vi "Perform Action.vi"(8 "error in (no error)":errorcluster, 10 "Input":variant, 11 "Sample PI Control in":refnum<class "Sample PI Control.lvclass">) -> (0 "error out":errorcluster, 2 "Output":variant, 3 "Sample PI Control out":refnum<class "Sample PI Control.lvclass">)   [LabVIEW 2023, in "Sample PI Control.lvclass"]
uses:
  Sample PI Control.lvclass
  D:/git/HAL/HAL GOOP4/Task/Task Base/Task Base.lvclass
  Task/Task Base/Task Base.lvclass/Task Base.ctl
  <vilib>/Utility/error.llb/Error Cluster From Error Code.vi
  <vilib>/addons/control/pid/pid.llb/PID (DBL).vi
  Sample PI Control.lvclass/Sample PI Control.ctl
  Measure and Stimulus Subsystems/Measure and Stimulus Subsystems.lvclass
  Task/Task Base/Task Base.lvclass
  <vilib>/addons/control/pid/NI_PID_pid.lvlib
panel:
  out "Powersensor Scalar":dbl
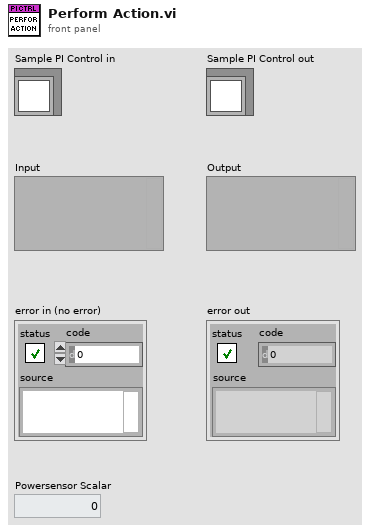
[diagram p1: front panel]
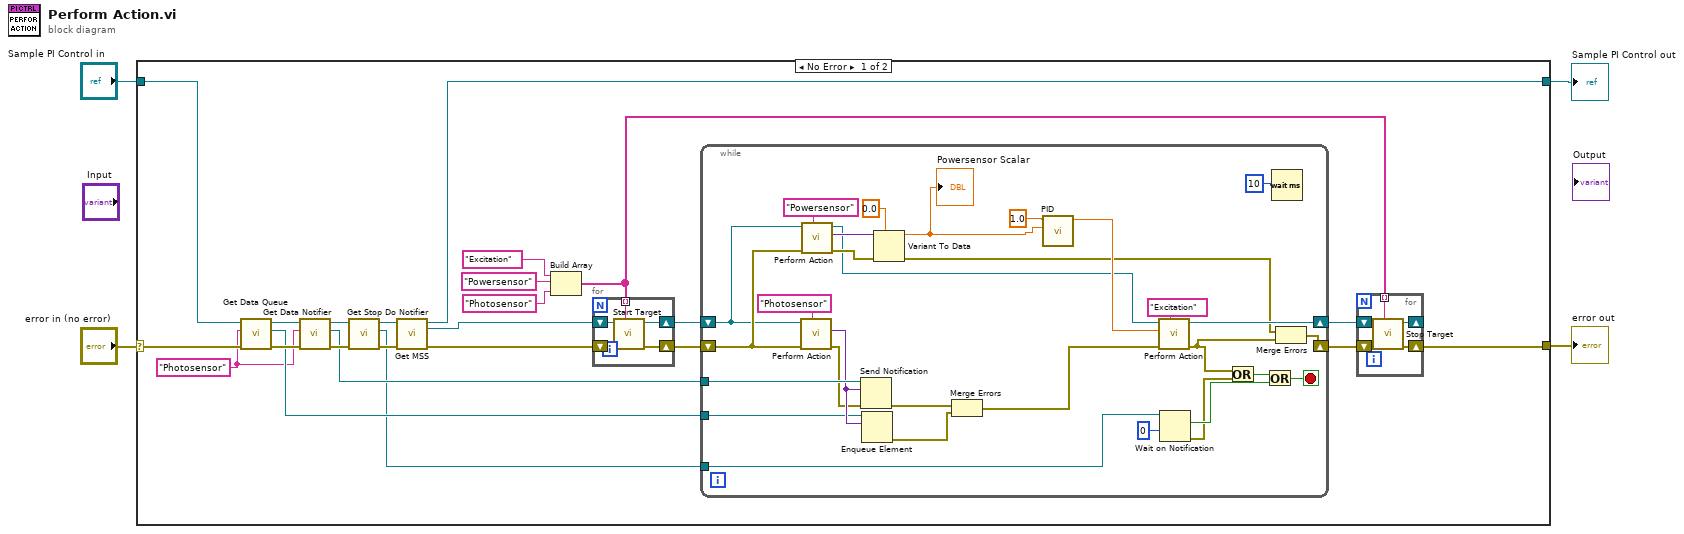
[diagram p0: block diagram]
diagram:
  n1 = case shown="No Error" "error in (no error)" {
    selector: "error in (no error)" -> [w25 w70]
    tunnel: [w21 w70] -> w3
    tunnel: [w11 w69] -> w1
    tunnel: "Sample PI Control in" -> [w13 w69]
    frame No Error {
      w7 = "Photosensor" ("Target Identifier")
      n2 = call "Get Data Queue.vi"("error in (no error)"=w25, "Target Name"=w7, "Task Base in"=w13) -> ("error out"=w14:errorcluster, "Data Queue"=w12:refnum<queue>, "Task Base out"=w9:refnum<class "Sample PI Control.lvclass">)  [unwired: 6 in]
      n3 = call "Get Data Notifier.vi"("error in (no error)"=w14, "Target Name"=w7, "Task Base in"=w9) -> ("error out"=w10:errorcluster, "Data Notifier"=w6:refnum<notifier>, "Task Base out"=w8:refnum<class "Sample PI Control.lvclass">)  [unwired: 6 in]
      n4 = call "Get Stop Do Notifier.vi"("error in (no error)"=w10, "Task Base in"=w8) -> ("error out"=w20:errorcluster, "Stop Do"=w5:refnum<notifier>, "Task Base out"=w19:refnum<class "Sample PI Control.lvclass">)  [unwired: 7 in]
      n5 = call "Get MSS.vi"("error in (no error)"=w20, "Task Base in"=w19) -> ("error out"=w24:errorcluster, "MSS"=w23:refnum<class "Measure and Stimulus Subsystems.lvclass">, "Task Base out"=w11:refnum<class "Sample PI Control.lvclass">)  [unwired: 7 in]
      n6 = Build Array("Excitation" ("Target Ident"), "Powersensor" ("Target Identifier"), "Photosensor" ("Target Identifier")) -> (w15:string[])
      n7 = for {
        shift-right: [w33] -> w28
        shift-left: w24 -> [w31]
        shift-right: [w32] -> w27
        shift-left: w23 -> [w30]
        tunnel: w15 -> [w29] mode=indexing
        n8 = call "Start Target.vi"("Target Ident"=w29, "Error In"=w31, "reference in"=w30) -> ("Error Out"=w33:errorcluster, "reference out"=w32:refnum<class "Measure and Stimulus Subsystems.lvclass">)  [unwired: 7 in]
      }
      n9 = while {
        shift-right: [w50] -> w26
        shift-left: w28 -> [w56]
        shift-right: [w58] -> w22
        shift-left: w27 -> [w55]
        tunnel: w6 -> [w45]
        tunnel: w12 -> [w40]
        tunnel: w5 -> [w34]
        stop <- w48 stop-if-true
        n10 = call "Perform Action.vi"("Target Ident"="Photosensor" ("Target Identifier"), "Error In"=w56, "reference in"=w55) -> ("Error Out"=w38:errorcluster, "Output"=w41:variant)  [unwired: 6 in, 1 out]
        n11 = call "Perform Action.vi"("Target Ident"="Powersensor" ("Target Identifier"), "Error In"=w56, "reference in"=w55) -> ("Error Out"=w61:errorcluster, "Output"=w60:variant, "reference out"=w51:refnum<class "Measure and Stimulus Subsystems.lvclass">)  [unwired: 6 in]
        n12 = Send Notification(notification=w41, notifier=w45, error in (no error)=w38) -> (error out=w36:errorcluster)  [unwired: 1 out]
        n13 = Enqueue Element(queue=w40, element=w41) -> (error out=w39:errorcluster)  [unwired: 2 in, 2 out]
        n14 = Variant To Data(error in=w61, type=0.0, Variant=w60) -> (data=w53:dbl, error out=w49:errorcluster)
        "Powersensor Scalar" <- w53
        n15 = Merge Errors(w36, w39) -> (w37:errorcluster)
        n16 = call-poly <vilib>:"PID.vi"("process variable"=w53, "setpoint"=1.0) -> ("output"=w52:dbl)  [unwired: 8 in, 1 out]
        n17 = call "Perform Action.vi"("Target Ident"="Excitation", "Error In"=w37, "Input"=w52, "reference in"=w51) -> ("Error Out"=w42:errorcluster, "reference out"=w58:refnum<class "Measure and Stimulus Subsystems.lvclass">)  [unwired: 5 in, 1 out]
        n18 = Wait on Notification(notifier=w34, timeout in ms (-1)=0) -> (notification=w46:bool, error out=w44:errorcluster)  [unwired: 2 in, 2 out]
        n19 = Or(x=w42, y=w44) -> (x .or. y?=w43:bool)
        n20 = Or(x=w43, y=w46) -> (x .or. y?=w48:bool)
        n21 = Wait (ms)(milliseconds to wait=u32 10) -> ()  [unwired: 1 out]
        n22 = Merge Errors(w49, w42) -> (w50:errorcluster)
      }
      n23 = for {
        shift-right: [w66] -> w21
        shift-left: w26 -> [w68]
        tunnel: w15 -> [w65] mode=indexing
        shift-right: [w64] -> _
        shift-left: w22 -> [w67]
        n24 = call "Stop Target.vi"("Target Ident"=w65, "Error In"=w68, "reference in"=w67) -> ("Error Out"=w66:errorcluster, "reference out"=w64:refnum<class "Measure and Stimulus Subsystems.lvclass">)  [unwired: 7 in]
      }
    }
    frame Error {
    }
  }
  "error out" <- w3
  "Sample PI Control out" <- w1
